vi "readChannelSystemMaxVolt.vi"(3 "error out 2":errorcluster caption="error out", 4 "通道号":i32, 5 "B3":i32, 6 "VISA resource name out 2":refnum<visa-resource-name>) -> (0 "error out":errorcluster, 1 "输出变量":dbl, 2 "VISA resource name out":refnum<visa-resource-name>)   [LabVIEW 2018]
panel:
  out "Serial Settings:Number of Bytes at Serial Port":u32
  out "返回数":u32
  out "添加的数组":u8[](array[numeric])
  out "输出变量 2":dbl
  out "子字符串":string
  out "字符串":string
  out "无符号字节数组":u8[](array[numeric])
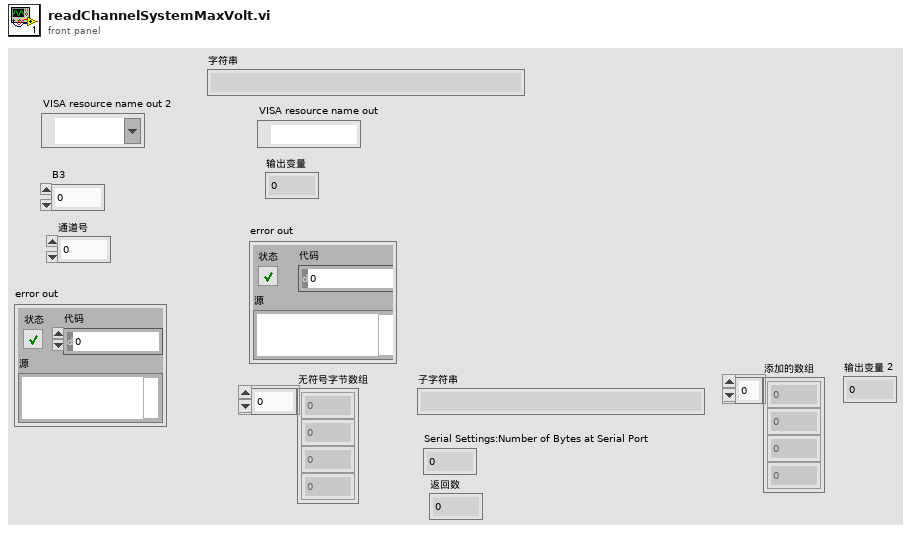
[diagram p1: front panel]
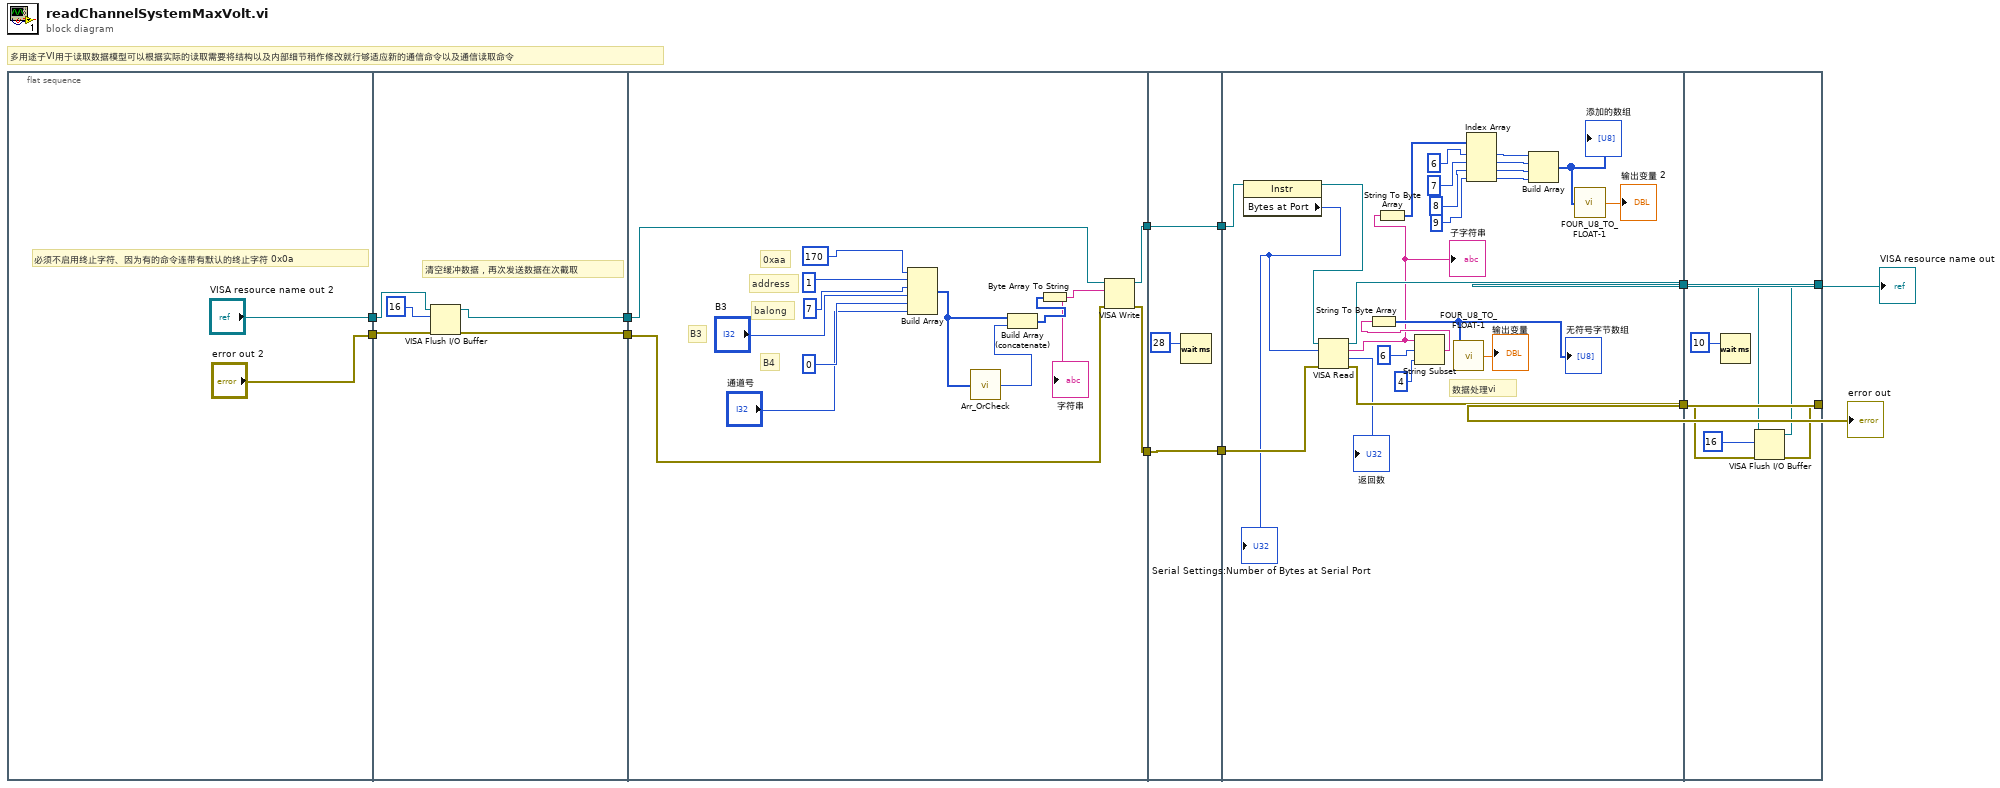
[diagram p0: block diagram]
diagram:
  # "多用途子VI用于读取数据模型可以根据实际的读取需要将结构以及内部细节稍作修改就行够适应新的通信命令以及通信读取命令"
  n1 = flat-sequence {
    tunnel: ["VISA resource name out 2"] -> w4
    tunnel: ["error out 2"] -> w3
    tunnel: w4 -> [w18]
    tunnel: w3 -> [w16]
    tunnel: [w15] -> w2
    tunnel: [w17] -> w1
    tunnel: [w27] -> w12
    tunnel: [w25] -> w10
    tunnel: w2 -> [w26]
    tunnel: w1 -> [w28]
    tunnel: w12 -> [w35]
    tunnel: [w35] -> w11
    tunnel: w10 -> [w34]
    tunnel: [w34] -> w9
    tunnel: w11 -> [w39]
    tunnel: w9 -> [w58]
    tunnel: [w57] -> w6
    tunnel: [w56] -> w5
    tunnel: [w62] -> w7
    tunnel: [w61] -> w8
    tunnel: w6 -> [w63]
    tunnel: w5 -> [w64]
    frame #0 {
      # "必须不启用终止字符、因为有的命令连带有默认的终止字符 0x0a"
    }
    frame #1 {
      # "清空缓冲数据，再次发送数据在次截取"
      n2 = VISA Flush I/O Buffer(VISA resource name=w18, mask (16)=16, error in (no error)=w16) -> (VISA resource name out=w17:refnum<visa-resource-name>, error out=w15:errorcluster)
    }
    frame #2 {
      # "B4"
      # "B3"
      # "balong"
      # "address"
      # "0xaa"
      n3 = Build Array(170, 1, 7, "B3", 0, "通道号") -> (w24:i32[])
      n4 = call "Arr_OrCheck.vi"("数组"=w24) -> ("抑或的数据值"=w23:u8)
      n5 = Build Array (concatenate)(w24, w23) -> (w22:i32[])
      n6 = Byte Array To String(unsigned byte array=w22) -> (string=w21:string)
      "字符串" <- w21
      n7 = VISA Write(VISA resource name=w28, write buffer=w21, error in (no error)=w26) -> (VISA resource name out=w27:refnum<visa-resource-name>, error out=w25:errorcluster)  [unwired: 1 out]
    }
    frame #3 {
      n8 = Wait (ms)(milliseconds to wait=28) -> ()  [unwired: 1 out]
    }
    frame #4 {
      # "数据处理vi"
      n9 = property class="Instr"(reference=w39) -> (reference out=w38:refnum<visa-resource-name>, "Bytes at Port"=w37:u32)  [unwired: 1 in, 1 out]
      "Serial Settings:Number of Bytes at Serial Port" <- w37
      n10 = VISA Read(VISA resource name=w38, byte count=w37, error in (no error)=w58) -> (VISA resource name out=w56:refnum<visa-resource-name>, read buffer=w41:string, return count=→"返回数":u32, error out=w57:errorcluster)
      "子字符串" <- w41
      n11 = String To Byte Array(string=w41) -> (unsigned byte array=w53:u8[])
      n12 = String Subset(string=w41, offset (0)=6 ("偏移量(0)"), length (rest)=4) -> (substring=w42:string)
      n13 = String To Byte Array(string=w42) -> (unsigned byte array=w60:u8[])
      "无符号字节数组" <- w60
      n14 = call "FOUR_U8_TO_FLOAT-1.vi"("接收数据4*U8"=w60) -> ("输出变量"=→"输出变量":dbl)
      n15 = Index Array(array=w53, index #1=6 ("偏移量(0)"), index #2=7 ("偏移量(0)"), index #3=8 ("偏移量(0)"), index #4=9 ("偏移量(0)")) -> (element #1=w48:u8, element #2=w47:u8, element #3=w46:u8, element #4=w45:u8)
      n16 = Build Array(w48, w47, w46, w45) -> (w44:u8[])
      "添加的数组" <- w44
      n17 = call "FOUR_U8_TO_FLOAT-1.vi"("接收数据4*U8"=w44) -> ("输出变量"=→"输出变量 2":dbl)
    }
    frame #5 {
      n18 = Wait (ms)(milliseconds to wait=10) -> ()  [unwired: 1 out]
      n19 = VISA Flush I/O Buffer(VISA resource name=w64, mask (16)=16, error in (no error)=w63) -> (VISA resource name out=w62:refnum<visa-resource-name>, error out=w61:errorcluster)
    }
  }
  "VISA resource name out" <- w7
  "error out" <- w8
